vi "replace array elements (mask).vi"(1 "input array of numbers":dbl[unit][](array[numeric]), 2 "array of booleans (mask)":bool[](array[boolean]), 3 "value":dbl[unit]) -> (0 "output array":dbl[unit][](array[numeric]))   [LabVIEW 2023]
doc: "Replaces all elements of numerical array that have \"true\" values in the corresponding mask, with \"value\"."
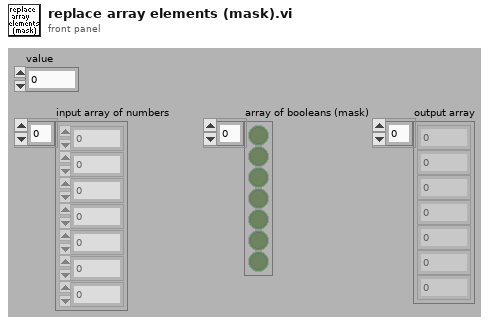
[diagram p1: front panel]
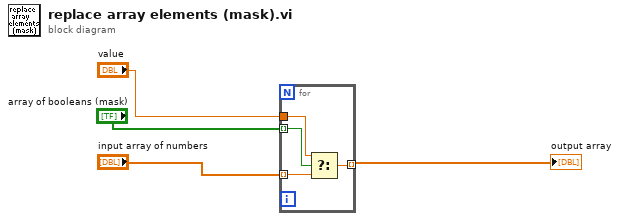
[diagram p0: block diagram]
diagram:
  n1 = for {
    tunnel: "array of booleans (mask)" -> [w8] mode=indexing
    tunnel: "input array of numbers" -> [w7] mode=indexing
    tunnel: [w6] -> w4 mode=indexing
    tunnel: "value" -> [w5]
    n2 = Select(t=w5, s=w8, f=w7) -> (s? t:f=w6:dbl[unit])
  }
  "output array" <- w4
